vi "Begin.vi"(11 "Image Size":T1=enum."160x120") -> (0 "error out":errorcluster)   [LabVIEW 2012]
doc: "Called before other user functions, this VI is expected to open initial I/O refnums, load in file data, and do all program initialization. Notice that the <B>error out</B> terminal is simply used for data flow. Wiring it to other structures or subVIs ensures that this VI runs first."
uses:
  <vilib>/Rock Robotics/SystemInterfaces/DIO/FPGA_DIOPWMChannel.ctl
  <vilib>/Rock Robotics/WPI/Camera/WPI_CameraWhite Balance Values.ctl
  <vilib>/Rock Robotics/WPI/Camera/WPI_CameraExposure Values.ctl
  <vilib>/Rock Robotics/WPI/Camera/WPI_CameraFrameRate.ctl
  <vilib>/Rock Robotics/WPI/SafetyOutput/WPI_SafetyOutputConfigMenu.ctl
  Robot Global Data.vi
  <vilib>/Rock Robotics/WPI/DriverStation/WPI_DriverStationRobotMode2.ctl
  <vilib>/Rock Robotics/WPI/Joystick/WPI_JoystickDeviceEnum.ctl
  <vilib>/Rock Robotics/WPI/Solenoid/WPI_SolenoidChannel.ctl
  <vilib>/Rock Robotics/SystemInterfaces/DIO/FPGA_DIORelayChannel.ctl
  <vilib>/Rock Robotics/SystemInterfaces/DIO/FPGA_DIOChannel.ctl
  <vilib>/Rock Robotics/WPI/Solenoid/WPI_SolenoidOpenDouble.vi
  <vilib>/Rock Robotics/WPI/RobotDrive/WPI_RobotDriveOpen2MotorWithTalon.vi
  <vilib>/Rock Robotics/SystemInterfaces/Typedef/FPGA_TypedefSolenoidModule.ctl
  <vilib>/Rock Robotics/WPI/Solenoid/WPI_SolenoidSetEnum.vi
  <vilib>/Rock Robotics/WPI/Solenoid/WPI_SolenoidValue.ctl
  <vilib>/Rock Robotics/WPI/MotorControl/WPI_MotorControlOpen Jaguar.vi
  <vilib>/Rock Robotics/SystemInterfaces/Typedef/FPGA_TypedefDigitalModule.ctl
  <vilib>/Rock Robotics/WPI/Camera/WPI_CameraImageSize.ctl
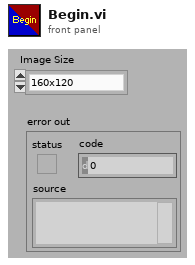
[diagram p1: front panel]
types:
  T1 = typedef "WPI_CameraImageSize.ctl" = enum16{"640x480", "320x240", "160x120"}
  T2 = typedef "FPGA_TypedefDigitalModule.ctl" = enum16{"Digital Module 1", "Digital Module 2"}
  T3 = typedef "WPI_SolenoidValue.ctl" = enum16{"Off", "On", "Forward", "Reverse"}
  T4 = typedef "FPGA_TypedefSolenoidModule.ctl" = enum16{"Solenoid Module 1", "Solenoid Module 2"}
  T5 = typedef "WPI_SolenoidChannel.ctl" = enum8{"Solenoid 1", "Solenoid 2", "Solenoid 3", "Solenoid 4", "Solenoid 5", "Solenoid 6", "Solenoid 7", "Solenoid 8", "Invalid"}
  T6 = typedef "FPGA_DIOChannel.ctl" = enum8{"DIO 1", "DIO 2", "DIO 3", "DIO 4", "DIO 5", "DIO 6", "DIO 7", "DIO 8", "DIO 9", "DIO 10", "DIO 11", "DIO 12", "DIO 13", "DIO 14", "Invalid"}
  T7 = typedef "FPGA_DIORelayChannel.ctl" = enum8{"Relay 1", "Relay 2", "Relay 3", "Relay 4", "Relay 5", "Relay 6", "Relay 7", "Relay 8", "Invalid"}
  T8 = typedef "WPI_JoystickDeviceEnum.ctl" = enum16{"USB 1", "USB 2", "USB 3", "USB 4", "Kinect 1", "Kinect 2"}
  T9 = typedef "WPI_DriverStationRobotMode2.ctl" = enum16{"Autonomous Disabled", "Autonomous Enabled", "Teleop Disabled", "Teleop Enabled", "Timeout", "Finish", "Test Disabled", "Test Enabled"}
  T10 = typedef "WPI_SafetyOutputConfigMenu.ctl" = enum16{"Enable", "Disable"}
  T11 = typedef "WPI_CameraFrameRate.ctl" = u32
  T12 = typedef "WPI_CameraExposure Values.ctl" = enum16{"Auto", "Flicker-free 50 Hz", "Flicker-free 60 Hz", "Hold current"}
  T13 = typedef "WPI_CameraWhite Balance Values.ctl" = enum16{"Auto", "Fixed indoor", "Fixed outdoor 1", "Fixed outdoor 2", "Fixed fluorescent 1", "Fixed fluorescent 2", "Hold current"}
  T14 = typedef "FPGA_DIOPWMChannel.ctl" = enum8{"PWM 1", "PWM 2", "PWM 3", "PWM 4", "PWM 5", "PWM 6", "PWM 7", "PWM 8", "PWM 9", "PWM 10", "Invalid"}
  T15 = typedef "WPI_SolenoidDevRef.ctl" = cluster{"DevStatus":errorcluster, "Solenoid Module":T4, "Forward Solenoid Channel":T5, "Reverse Solenoid Channel":T5}
  T16 = typedef "WPI_CameraDevRef.ctl" = cluster{"Camera Address":string, "CameraStatus":errorcluster, "Acquire Image Notifier":refnum<notifier>}
  T17 = typedef "WPI_RobotDriveDevRef.ctl" = cluster{"DevStatus":errorcluster, "Motors[]":T18[], "Square Inputs":bool, "Max Output":dbl, "Isochronous":bool}
  T18 = typedef "WPI_MotorControlDeviceRef.ctl" = cluster{"DeviceStatus":errorcluster, "Type":enum16{"PWM", "CAN"}, "PWM":cluster{"Digital Module":T2, "PWM Channel":T14, "DeadBand":T19}, "CAN":cluster{"Device Number":u8, "Control Mode":T20, "Semaphore":T21, "Max Vout":dbl}, "Invert":bool, "TransformRef":T22, "InvTransformRef":T22}
  T19 = typedef "WPI_PWMDeadband.ctl" = cluster{"Name":string, "maxPositivePwm":i32, "minPositivePwm":i32, "centerPwm":i32, "maxNegativePwm":i32, "minNegativePwm":i32, "angularRange":u16}
  T20 = typedef "WPI_CANJaguar_ControlMode.ctl" = enum8{"Percent VBus", "Current", "Speed", "Position", "Voltage"}
  T21 = typedef "Semaphore RefNum" = refnum<k1>
  T22 = typedef "WPI_PWMTransform_ConPane.ctl" = refnum<vi>
  T23 = typedef "WPI_JoystickDevRef.ctl" = cluster{"Device":T8}
  T24 = typedef "WPI_CompressorDevRef.ctl" = cluster{"DevStatus":errorcluster, "DigitalInputDevRef":T25, "RelayDevRef":T26}
  T25 = typedef "WPI_DigitalInputDevRef.ctl" = cluster{"DevStatus":errorcluster, "DIO Channel":T6, "Digital Module":T2}
  T26 = typedef "WPI_RelayDevRef.ctl" = cluster{"DevStatus":errorcluster, "Relay Channel":T7, "Digital Module":T2, "Relay Direction":T27}
  T27 = typedef "WPI_RelayDirection.ctl" = enum16{"Both directions", "Forward only", "Reverse only"}
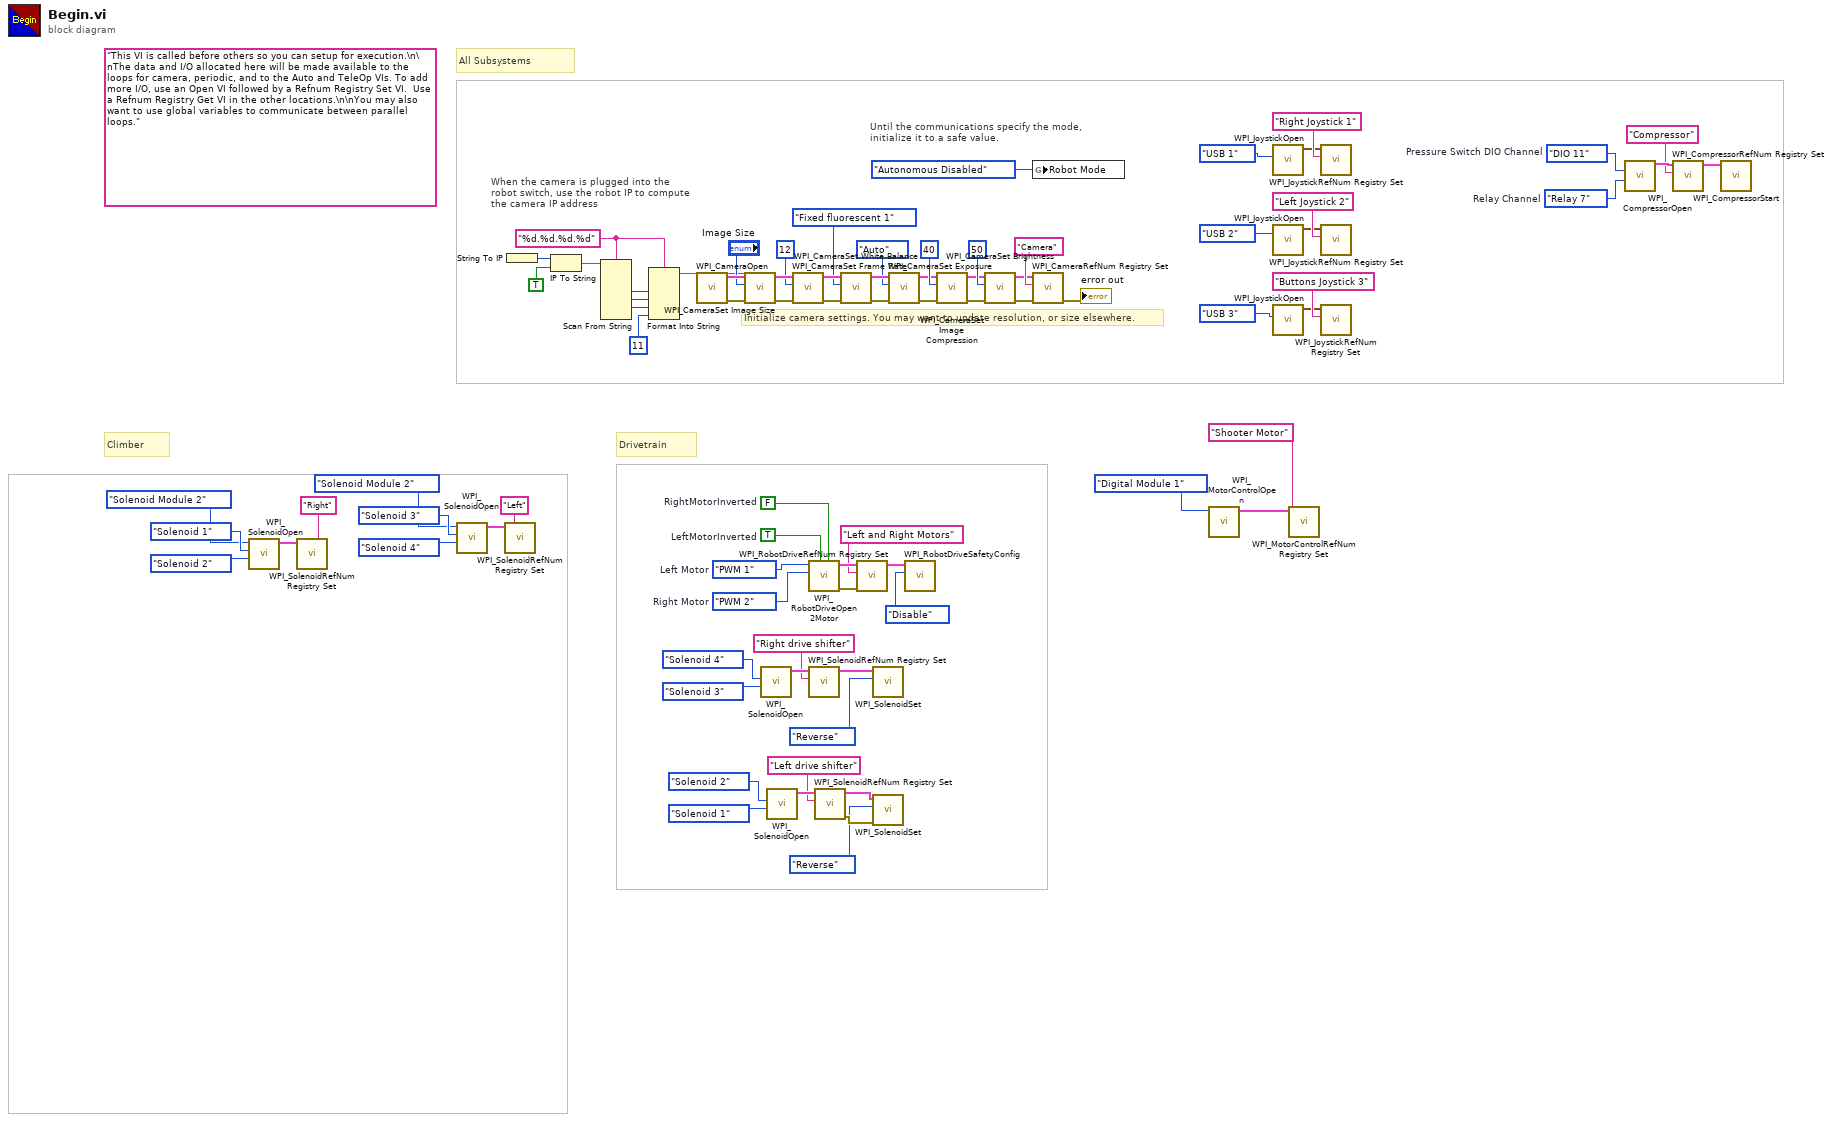
[diagram p0: block diagram]
diagram:
  w28 = FPGA_DIOChannel."DIO 11"  # Pressure Switch DIO Channel
  w31 = FPGA_DIORelayChannel."Relay 7"  # Relay Channel
  w46 = "%d.%d.%d.%d" ("format string")
  (unwired) "This VI is called before others so you can setup for execution.\n\nThe data and I/O allocated here will be made available to the loops for camera, periodic, and to the Auto and TeleOp VIs. To add more I/O, use an Open VI followed by a Refnum Registry Set VI.  Use a Refnum Registry Get VI in the other locations.\n\nYou may also want to use global variables to communicate between parallel loops."
  w57 = FPGA_DIOPWMChannel."PWM 2"  # Right Motor
  w58 = FPGA_DIOPWMChannel."PWM 1"  # Left Motor
  w80 = TRUE  # LeftMotorInverted
  w81 = FALSE  # RightMotorInverted
  # "All Subsystems"
  # "Climber"
  # "Drivetrain"
  # "Until the communications specify the mode,\ninitialize it to a safe value."
  # "When the camera is plugged into the\nrobot switch, use the robot IP to compute\nthe camera IP address"
  # "Initialize camera settings. You may want to update resolution, or size elsewhere."
  n1 = call-poly <vilib>:"WPI_SolenoidOpen.vi"("Reverse Solenoid Channel"=WPI_SolenoidChannel."Solenoid 2", "Forward Solenoid Channel"=WPI_SolenoidChannel."Solenoid 1", "Solenoid Module (Module 1)"=FPGA_TypedefSolenoidModule."Solenoid Module 2") -> ("SolenoidDevRef"=w13:T15)  [unwired: 7 in, 1 out]
  n2 = call <vilib>:"WPI_SolenoidRefNum Registry Set.vi"("refnum name"="Right", "SolenoidDevRef"=w13) -> ()  [unwired: 8 in, 2 out]
  n3 = call-poly <vilib>:"WPI_SolenoidOpen.vi"("Reverse Solenoid Channel"=WPI_SolenoidChannel."Solenoid 4", "Forward Solenoid Channel"=WPI_SolenoidChannel."Solenoid 3", "Solenoid Module (Module 1)"=FPGA_TypedefSolenoidModule."Solenoid Module 2") -> ("SolenoidDevRef"=w18:T15)  [unwired: 7 in, 1 out]
  n4 = call <vilib>:"WPI_SolenoidRefNum Registry Set.vi"("refnum name"="Left", "SolenoidDevRef"=w18) -> ()  [unwired: 8 in, 2 out]
  n5 = String To IP() -> (0:w53:u32)  [unwired: 1 in]
  n6 = IP To String(1:TRUE ("dot notation? (F)"), 2:w53) -> (0:w51:string)
  n7 = Scan From String(format string=w46, input string=w51) -> (output 1=w50:i32, output 2=w49:i32, output 3=w48:i32)  [unwired: 7 in, 3 out]
  n8 = Format Into String(format string=w46, w50, w49, w48, 11 ("Compression")) -> (resulting string=w42:string)  [unwired: 2 in, 1 out]
  n9 = call <vilib>:"WPI_CameraOpen.vi"("Camera Address"=w42) -> ("error out"=w67:errorcluster, "CameraDevRef"=w68:T16)  [unwired: 1 in, 8 out]
  n10 = call <vilib>:"WPI_CameraSet Image Size.vi"("error in (no error)"=w67, "Image Size"="Image Size", "CameraDevRef"=w68) -> ("error out"=w66:errorcluster, "CameraDevRef Out"=w69:T16)  [unwired: 7 out]
  n11 = call-poly <vilib>:"WPI_SolenoidOpen.vi"("Reverse Solenoid Channel"=WPI_SolenoidChannel."Solenoid 3", "Forward Solenoid Channel"=WPI_SolenoidChannel."Solenoid 4") -> ("SolenoidDevRef"=w22:T15)  [unwired: 8 in, 1 out]
  n12 = call-poly <vilib>:"WPI_SolenoidOpen.vi"("Reverse Solenoid Channel"=WPI_SolenoidChannel."Solenoid 1", "Forward Solenoid Channel"=WPI_SolenoidChannel."Solenoid 2") -> ("SolenoidDevRef"=w26:T15)  [unwired: 8 in, 1 out]
  n13 = call <vilib>:"WPI_CameraSet Frame Rate.vi"("error in (no error)"=w66, "Frame Rate (fps)"=T11 12, "CameraDevRef"=w69) -> ("error out"=w65:errorcluster, "CameraDevRef Out"=w71:T16)  [unwired: 7 out]
  n14 = call-poly <vilib>:"WPI_RobotDriveOpen2Motor.vi"("Right Motor Inverted"=w81, "Left Motor Inverted"=w80, "Right Motor"=w57, "Left Motor"=w58) -> ("error out"=w76:errorcluster, "RobotDriveDevRef"=w78:T17)  [unwired: 1 in, 5 out]
  n15 = call <vilib>:"WPI_SolenoidRefNum Registry Set.vi"("refnum name"="Right drive shifter", "SolenoidDevRef"=w22) -> ("SolenoidDevRef"=w8:T15)  [unwired: 8 in, 1 out]
  n16 = call <vilib>:"WPI_SolenoidRefNum Registry Set.vi"("refnum name"="Left drive shifter", "SolenoidDevRef"=w26) -> ("error out"=w6:errorcluster, "SolenoidDevRef"=w7:T15)  [unwired: 8 in]
  n17 = call <vilib>:"WPI_CameraSet White Balance.vi"("error in (no error)"=w65, "White Balance"=WPI_CameraWhite_Balance_Values."Fixed fluorescent 1", "CameraDevRef"=w71) -> ("error out"=w64:errorcluster, "CameraDevRef Out"=w70:T16)  [unwired: 7 out]
  n18 = call <vilib>:"WPI_RobotDriveRefNum Registry Set.vi"("error in (no error)"=w76, "refnum name"="Left and Right Motors", "RobotDriveDevRef"=w78) -> ("RobotDriveDevRef"=w45:T17)  [unwired: 8 out]
  n19 = call-poly <vilib>:"WPI_SolenoidSet.vi"("Value"=WPI_SolenoidValue."Reverse", "SolenoidDevRef"=w8) -> ()  [unwired: 8 in, 2 out]
  n20 = call-poly <vilib>:"WPI_SolenoidSet.vi"("error in (no error)"=w6, "Value"=WPI_SolenoidValue."Reverse", "SolenoidDevRef"=w7) -> ()  [unwired: 7 in, 2 out]
  n21 = call <vilib>:"WPI_CameraSet Exposure.vi"("error in (no error)"=w64, "Exposure"=WPI_CameraExposure_Values."Auto", "CameraDevRef"=w70) -> ("error out"=w63:errorcluster, "CameraDevRef Out"=w73:T16)  [unwired: 7 out]
  n22 = call <vilib>:"WPI_RobotDriveSafetyConfig.vi"("mode"=WPI_SafetyOutputConfigMenu."Disable", "RobotDriveDevRef"=w45) -> ()  [unwired: 8 in, 2 out]
  n23 = call <vilib>:"WPI_CameraSet Image Compression.vi"("error in (no error)"=w63, "Compression"=40, "CameraDevRef"=w73) -> ("error out"=w62:errorcluster, "CameraDevRef Out"=w72:T16)  [unwired: 7 out]
  n24 = call <vilib>:"WPI_CameraSet Brightness.vi"("error in (no error)"=w62, "Brightness"=50, "CameraDevRef"=w72) -> ("error out"=w60:errorcluster, "CameraDevRef Out"=w61:T16)  [unwired: 7 out]
  n25 = global write "Robot Global Data.vi" "Robot Mode"(WPI_DriverStationRobotMode2."Autonomous Disabled" ("Robot Mode")) -> ()
  n26 = call <vilib>:"WPI_CameraRefNum Registry Set.vi"("error in (no error)"=w60, "refnum name"="Camera", "CameraDevRef"=w61) -> ("error out"=→"error out":errorcluster)  [unwired: 8 out]
  n27 = call-poly <vilib>:"WPI_MotorControlOpen.vi"("Digital Module (Module 1)"=FPGA_TypedefDigitalModule."Digital Module 1") -> ("MotorControlDeviceRef"=w3:T18)  [unwired: 9 in, 1 out]
  n28 = call <vilib>:"WPI_JoystickOpen.vi"("JoystickDevice"=WPI_JoystickDeviceEnum."USB 1") -> ("JoystickDevRef"=w40:T23)  [unwired: 10 in]
  n29 = call <vilib>:"WPI_JoystickOpen.vi"("JoystickDevice"=WPI_JoystickDeviceEnum."USB 2") -> ("JoystickDevRef"=w36:T23)  [unwired: 10 in]
  n30 = call <vilib>:"WPI_JoystickOpen.vi"("JoystickDevice"=WPI_JoystickDeviceEnum."USB 3") -> ("JoystickDevRef"=w33:T23)  [unwired: 10 in]
  n31 = call <vilib>:"WPI_MotorControlRefNum Registry Set.vi"("refnum name"="Shooter Motor", "MotorControlDevRef"=w3) -> ()  [unwired: 8 in, 2 out]
  n32 = call <vilib>:"WPI_JoystickRefNum Registry Set.vi"("refnum name"="Right Joystick 1", "JoystickDevRef"=w40) -> ()  [unwired: 8 in, 2 out]
  n33 = call <vilib>:"WPI_JoystickRefNum Registry Set.vi"("refnum name"="Left Joystick 2", "JoystickDevRef"=w36) -> ()  [unwired: 8 in, 2 out]
  n34 = call <vilib>:"WPI_JoystickRefNum Registry Set.vi"("refnum name"="Buttons Joystick 3", "JoystickDevRef"=w33) -> ()  [unwired: 8 in, 2 out]
  n35 = call <vilib>:"WPI_CompressorOpen.vi"("Pressure Switch DIO Channel"=w28, "Relay Channel"=w31) -> ("CompressorDevRef"=w30:T24)  [unwired: 12 in, 1 out]
  n36 = call <vilib>:"WPI_CompressorRefNum Registry Set.vi"("refnum name"="Compressor", "CompressorDevRef"=w30) -> ("CompressorDevRef"=w27:T24)  [unwired: 8 in, 1 out]
  n37 = call <vilib>:"WPI_CompressorStart.vi"("CompressorDevRef"=w27) -> ()  [unwired: 9 in, 2 out]
